vi "GetLevel1.vi"(8 "error in (no error)":errorcluster, 11 "TheConsumer in":refnum<class "TheConsumer.lvclass">) -> (0 "error out":errorcluster, 1 "Level2Class out":refnum<class "Level2Class.lvclass">, 3 "TheConsumer out":refnum<class "TheConsumer.lvclass">)   [LabVIEW 2019, in "TheConsumer.lvlib" / "TheConsumer.lvclass"]
uses:
  TheConsumer.lvclass
  Level2Class/Level2Class.lvclass
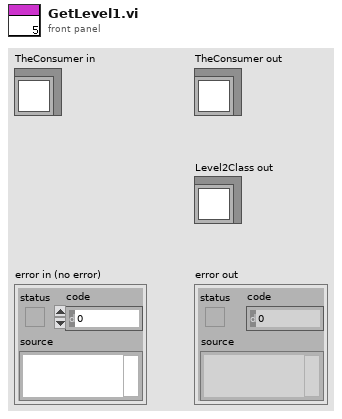
[diagram p1: front panel]
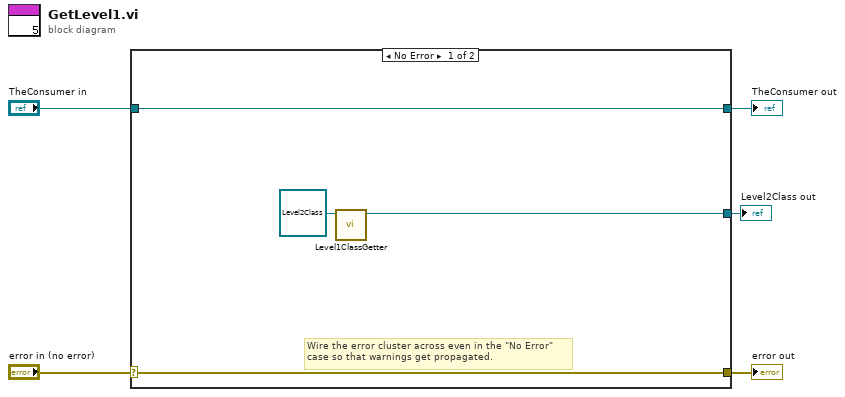
[diagram p0: block diagram]
diagram:
  n1 = case shown="No Error" "error in (no error)" {
    selector: "error in (no error)" -> [w8 w11]
    tunnel: [w8 w11] -> w4
    tunnel: [w9 w10] -> w2
    tunnel: "TheConsumer in" -> [w9 w10]
    tunnel: [w6 _] -> w1
    frame No Error {
      # "Wire the error cluster across even in the \"No Error\"\ncase so that warnings get propagated."
      n2 = call-dynamic "Level1ClassGetter.vi"("Level2Class in"=refnum<class "Level2Class.lvclass"> refnum) -> ("Level2Class out"=w6:refnum<class "Level2Class.lvclass">)  [unwired: 8 in, 2 out]
    }
    frame Error {
    }
  }
  "error out" <- w4
  "TheConsumer out" <- w2
  "Level2Class out" <- w1
